vi "LogIn.vi"() -> ()   [LabVIEW 2020]
panel:
  in  "Login":bool
  in  "Password":string
  in  "User Name":string
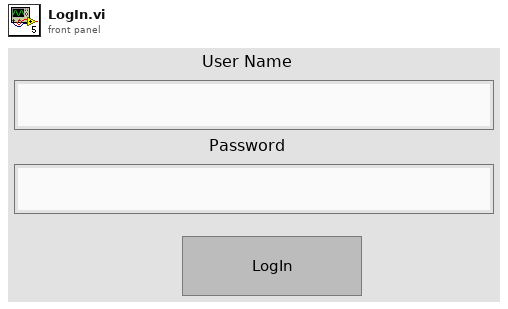
[diagram p1: front panel]
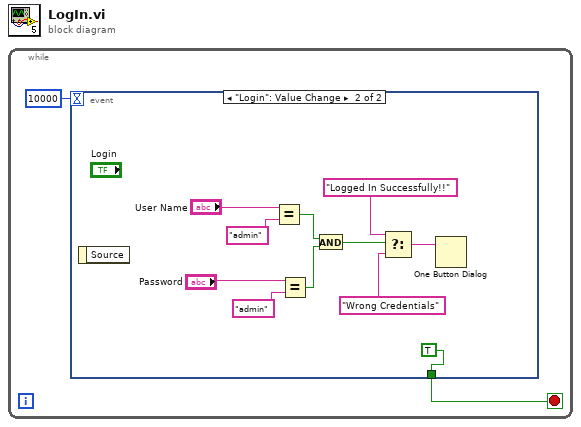
[diagram p0: block diagram]
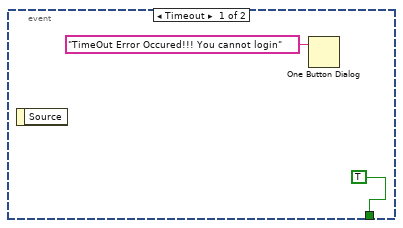
[diagram p2: hidden frame]
diagram:
  n1 = while {
    stop <- w2 stop-if-true
    n2 = event shown="[1] \"Login\": Value Change" {
      selector: _ -> [_ _]
      dyn-events: _ -> [_ _]
      timeout: 10000 -> [_ _]
      tunnel: [TRUE TRUE] -> w2
      event Timeout {
        n3 = event-data() -> ()  [unwired: 1 in, 1 out]
        n4 = One Button Dialog(message="TimeOut Error Occured!!! You cannot login") -> ()  [unwired: 1 in, 1 out]
      }
      event "Login": Value Change {
        n5 = event-data() -> ()  [unwired: 1 in, 1 out]
        n6 = Equal?(x="User Name", y="admin") -> (x = y?=w11:bool)
        n7 = Equal?(x="Password", y="admin") -> (x = y?=w10:bool)
        n8 = And(x=w11, y=w10) -> (x .and. y?=w9:bool)
        n9 = Select(t="Logged In Successfully!!", s=w9, f="Wrong Credentials") -> (s? t:f=w6:string)
        n10 = One Button Dialog(message=w6) -> ()  [unwired: 1 in, 1 out]
      }
    }
  }
